vi "DeregDataChannel.vi"(0 "channel":T1=1 items=["Channel 0", "Channel 1", "Channel 2", "Channel 3", "Channel 4", "Channel 5", "Channel 6", "Channel 7", "Channel 8", "Channel 9", "Channel 10", "Channel 11", "Channel 12", "Channel 13"], 5 "error in":T2) -> (19 "error out":T2)   [LabVIEW 2016]
doc: "By calling this vi the data reception into the buffer for the specified 'channel' is stopped. This prevents the buffer from consuming more and more memory."
uses:
  Controls/Error_Out.ctl
  Controls/Channel_Selection.ctl
  Files_ASC500/DLL/ASC500_RemoteControlV27.dll
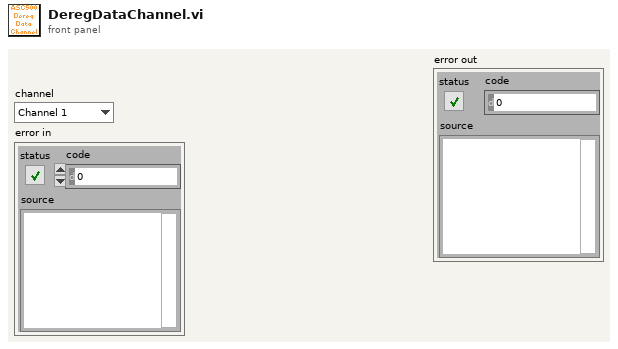
[diagram p1: front panel]
types:
  T1 = typedef "Channel_Selection.ctl" = i32
  T2 = typedef "Error_Out.ctl" = errorcluster
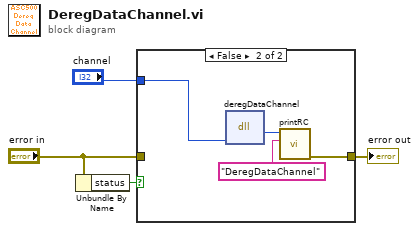
[diagram p0: block diagram]
diagram:
  n1 = Unbundle By Name("error in") -> ("status"=w4:bool)
  n2 = case shown="False" w4 {
    tunnel: "channel" -> [_ w9]
    tunnel: "error in" -> [w5 _]
    tunnel: [w5 w6] -> w1
    frame True {
    }
    frame False {
      n3 = dll-call lib="G:/SCMOperations/Share/ELE/Produkt Information/ASC500/04 Remote Control/02 development versions/2018Nov06/Files_ASC500/DLL/ASC500_RemoteControlV27.dll" fn="deregDataChannel"("Channel"=w9) -> ("return type"=w8:i32)  [unwired: 4 in, 2 out]
      n4 = call "printRC.vi"("additional information"="DeregDataChannel", "RC"=w8) -> ("error out"=w6:T2)  [unwired: 9 in]
    }
  }
  "error out" <- w1
